vi "Magnet Limits.vi"(0 "instrument.PPMS3":refnum<class "instrument.PPMS3.lvclass">, 5 "Helium (%)":dbl, 7 "Target Field (Oe)":dbl, 9 "Mode":T1, 11 "error in (no error)":errorcluster) -> (4 "instrument.PPMS3 out":refnum<class "instrument.PPMS3.lvclass">, 8 "Limited Field (Oe)":dbl, 10 "Mode out":T1, 15 "error out":errorcluster)   [LabVIEW 2019, in "instrument.PPMS3.lvclass"]
uses:
  instrument.PPMS3.lvclass
  <userlib>/LevyLab/Levylab Instruments/Instrument Types/Cryostat/Typedefs/Magnet Mode--Enum.ctl
  <userlib>/LevyLab/Levylab Instruments/Instrument Types/Cryostat/Instrument.Cryostat.lvclass
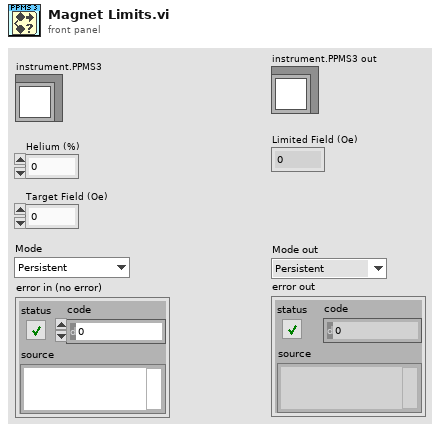
[diagram p1: front panel]
types:
  T1 = typedef "Instrument.Cryostat.lvclass/Magnet Mode--Enum.ctl" = enum16{"Persistent", "Driven"}
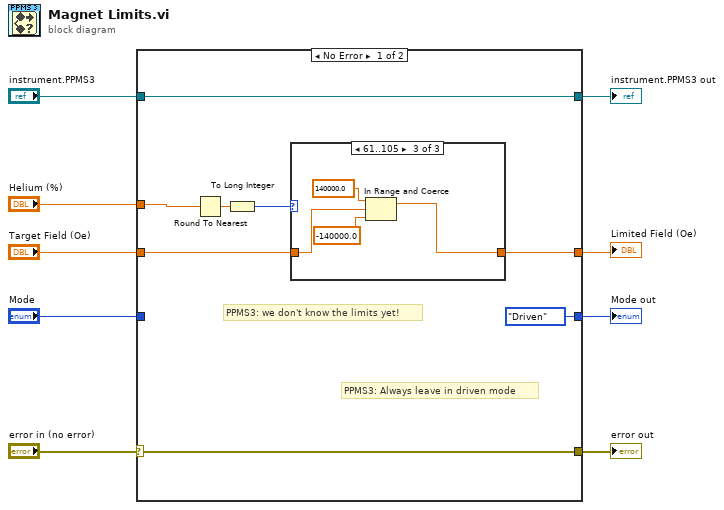
[diagram p0: block diagram]
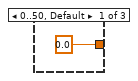
[diagram p2: hidden frame]
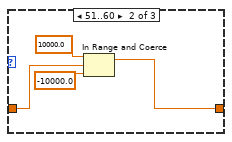
[diagram p3: hidden frame]
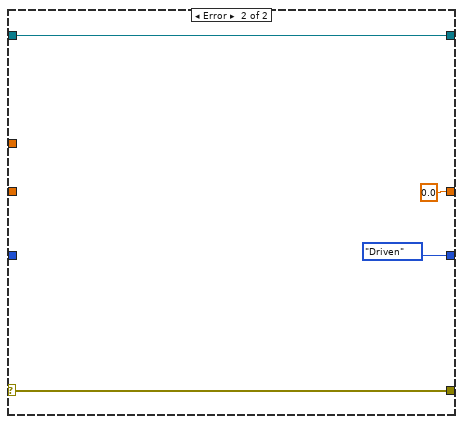
[diagram p4: hidden frame]
diagram:
  n1 = case shown="No Error" "error in (no error)" {
    selector: "error in (no error)" -> [w16 w30]
    tunnel: "Target Field (Oe)" -> [w13 _]
    tunnel: [w12 0.0 ("upper limit")] -> w3
    tunnel: "instrument.PPMS3" -> [w17 w29]
    tunnel: [w17 w29] -> w8
    tunnel: [w16 w30] -> w7
    tunnel: [Magnet_Mode--Enum."Driven" ("Mode") Magnet_Mode--Enum."Driven" ("Mode")] -> w2
    tunnel: "Mode" -> [_ _]
    tunnel: "Helium (%)" -> [w11 _]
    frame No Error {
      # "PPMS3: Always leave in driven mode"
      # "PPMS3: we don't know the limits yet!"
      n2 = Round To Nearest(number=w11) -> (nearest integer value=w15:dbl)
      n3 = To Long Integer(number=w15) -> (32bit integer=w14:i32)
      n4 = case shown="61..105" w14 {
        tunnel: w13 -> [_ w22 w26]
        tunnel: [0.0 ("upper limit") w19 w24] -> w12
        frame 0..50, Default {
        }
        frame 51..60 {
          n5 = In Range and Coerce(upper limit=10000.0, x=w22, lower limit=-10000.0) -> (coerced(x)=w19:dbl)  [unwired: 1 out]
        }
        frame 61..105 {
          n6 = In Range and Coerce(upper limit=140000.0, x=w26, lower limit=-140000.0) -> (coerced(x)=w24:dbl)  [unwired: 1 out]
        }
      }
    }
    frame Error {
    }
  }
  "Limited Field (Oe)" <- w3
  "instrument.PPMS3 out" <- w8
  "Mode out" <- w2
  "error out" <- w7
